vi "Delta_P.vi"() -> (0 "New Values In":string[][](array[string])=[["Test data5"]], 1 "New Chs In":string[](array[string])=["30-10-03:New:Channel new5"])   [LabVIEW 2021]
uses:
  Results_plotter_Global.vi
  Data plotting/subVIs/Plot_Values_Global.vi
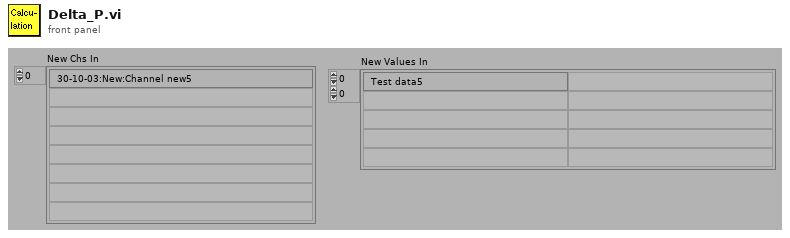
[diagram p1: front panel]
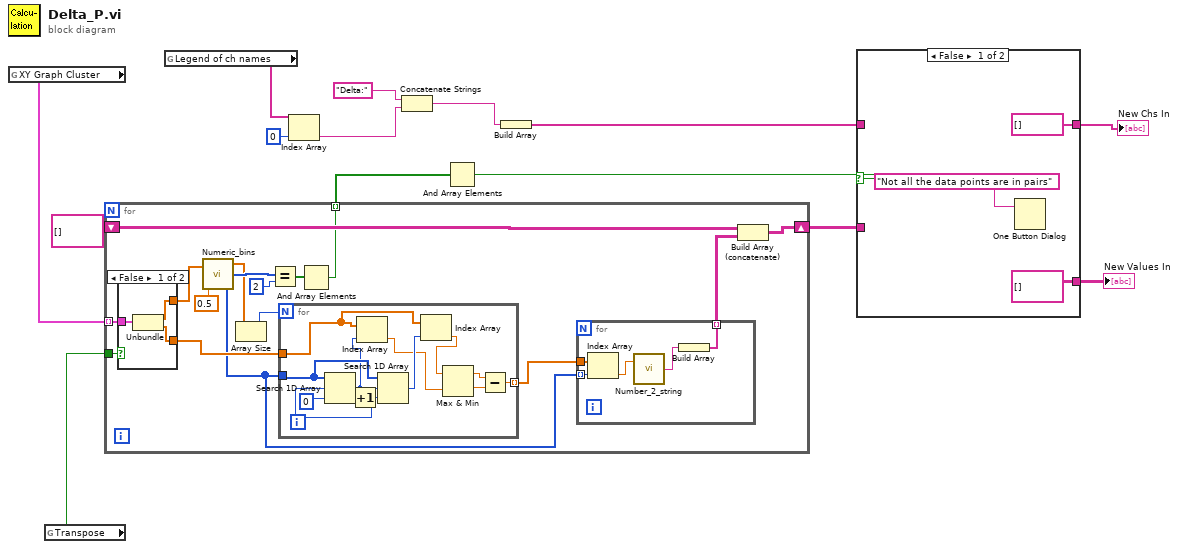
[diagram p0: block diagram]
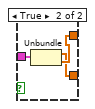
[diagram p3: hidden frame]
diagram:
  n1 = global read "Plot_Values_Global.vi" "XY Graph Cluster"() -> (w1:cluster{dbl[], dbl[]}[])
  n2 = global read "Results_plotter_Global.vi" "Transpose"() -> (w2:bool)
  n3 = for {
    tunnel: w1 -> [w30] mode=indexing
    shift-right: [w27] -> w3
    shift-left: string[][] [] -> [w29]
    tunnel: [w16] -> w8 mode=indexing
    tunnel: w2 -> [w15]
    n4 = case shown="False" w15 {
      tunnel: w30 -> [w33 w36]
      tunnel: [w32 w35] -> w26
      tunnel: [w31 w34] -> w19
      frame False {
        n5 = Unbundle(w33) -> (w32:dbl[], w31:dbl[])
      }
      frame True {
        n6 = Unbundle(w36) -> (w34:dbl[], w35:dbl[])
      }
    }
    n7 = call "Numeric_bins.vi"("Values"=w26, "Tolerance"=0.5) -> ("Bin Centres"=w21:dbl[], "No of points in bins"=w24:i32[], "Bin Index"=w18:i32[])
    n8 = Array Size(array=w21) -> (size(s)=w20:i32)
    n9 = Equal?(x=w24, y=2) -> (x = y?=w22:bool[])
    n10 = for {
      N: w20 -> [_]
      tunnel: w18 -> [w47]
      tunnel: w19 -> [w43]
      tunnel: [w38] -> w17 mode=indexing
      i -> [w46]
      n11 = Search 1D Array(1D array=w47, element=w46, start index (0)=0) -> (index of element=w45:i32)
      n12 = Increment(x=w45) -> (x+1=w37:i32)
      n13 = Index Array(array=w43, index=w45) -> (element=w41:dbl)
      n14 = Search 1D Array(1D array=w47, element=w46, start index (0)=w37) -> (index of element=w44:i32)
      n15 = Index Array(array=w43, index=w44) -> (element=w42:dbl)
      n16 = Max & Min(x=w42, y=w41) -> (max(x,y)=w39:dbl, min(x,y)=w40:dbl)
      n17 = Subtract(x=w39, y=w40) -> (x-y=w38:dbl)
    }
    n18 = And Array Elements(Boolean array=w22) -> (logical AND=w16:bool)
    n19 = for {
      tunnel: [w52] -> w28 mode=indexing
      tunnel: w18 -> [w51] mode=indexing
      tunnel: w17 -> [w50]
      n20 = Index Array(array=w50, index=w51) -> (element=w49:dbl)
      n21 = call "Number_2_string.vi"("number"=w49) -> ("String"=w53:string)  [unwired: 1 in]
      n22 = Build Array(w53) -> (w52:string[])
    }
    n23 = Build Array (concatenate)(w29, w28) -> (w27:string[][])
  }
  n24 = global read "Results_plotter_Global.vi" "Legend of ch names"() -> (w13:string[])
  n25 = Index Array(array=w13, index=0) -> (element=w9:string)
  n26 = Concatenate Strings("Delta:" ("string"), w9) -> (w11:string)
  n27 = And Array Elements(Boolean array=w8) -> (logical AND=w7:bool)
  n28 = Build Array(w11) -> (w5:string[])
  n29 = case shown="False" w7 {
    tunnel: [string[] [] w58] -> w6
    tunnel: w5 -> [_ w58]
    tunnel: [string[][] [] w57] -> w4
    tunnel: w3 -> [_ w57]
    frame False {
      n30 = One Button Dialog(message="Not all the data points are in pairs") -> ()  [unwired: 1 in, 1 out]
    }
    frame True {
    }
  }
  "New Chs In" <- w6
  "New Values In" <- w4
